vi "Outer Core.vi"   [LabVIEW 2015]
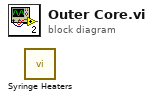
[diagram p0: block diagram]
diagram:
  n1 = call "Syringe Heaters.vi"() -> ()  [unwired: 12 in]
